vi "Maintain Loop Speed.vi"(7 "PID":T1={"proportional gain (Kc)"=10.0, "integral time (Ti, min)"=10.0, "derivative time (Td, min)"=0.0001}, 9 "setpoint (msec)":i32=25) -> (1 "Loop Time":dbl format="%0.2f")   [LabVIEW 2020]
uses:
  <vilib>/addons/control/pid/pid.llb/PID (DBL).vi
  <vilib>/ptbypt/NI_PtbyPt.lvlib
  <vilib>/addons/control/pid/NI_PID_pid.lvlib
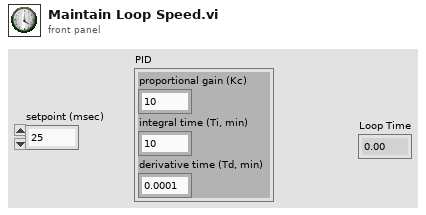
[diagram p1: front panel]
types:
  T1 = cluster{"proportional gain (Kc)":dbl, "integral time (Ti, min)":dbl, "derivative time (Td, min)":dbl}
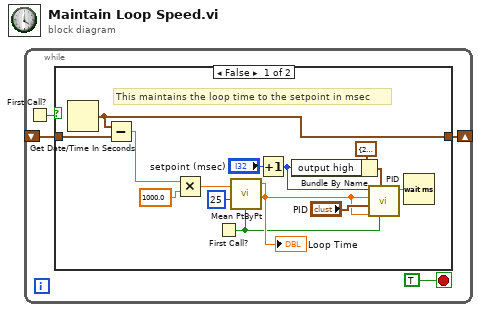
[diagram p0: block diagram]
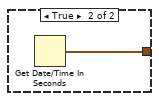
[diagram p2: hidden frame]
diagram:
  n1 = while {
    shift-right: [w2] -> _
    shift-left: _ -> [w3]
    stop <- TRUE stop-if-true
    n2 = First Call?() -> (First Call?: T/F=w1:bool)
    n3 = case shown="False" w1 {
      tunnel: w3 -> [w8 _]
      tunnel: [w7 w19] -> w2
      frame False {
        # "This maintains the loop time to the setpoint in msec"
        n4 = Get Date/Time In Seconds() -> (seconds since 1Jan1904=w7:timestamp)
        n5 = Subtract(x=w7, y=w8) -> (x-y=w6:dbl)
        n6 = Multiply(x=w6, y=1000.0) -> (x*y=w14:dbl)
        n7 = First Call?() -> (First Call?: T/F=w12:bool)
        n8 = call <vilib>:"Mean PtByPt.vi"("x"=w14, "sample length"=25, "initialize"=w12) -> ("mean"=w13:dbl)  [unwired: 1 in, 1 out]
        "Loop Time" <- w13
        n9 = Increment(x="setpoint (msec)") -> (x+1=w5:i32)
        n10 = Bundle By Name(cluster=cluster{"output high":dbl, "output low":dbl} {"output high"=25.0, "output low"=0.0} ("output range"), "output high"=w5) -> (w9:cluster{"output high":dbl, "output low":dbl})
        n11 = call-poly <vilib>:"PID.vi"("reinitialize? (F)"=w12, "output range"=w9, "dt (s)"=w13, "PID gains"="PID", "process variable"=w13, "setpoint"=w5) -> ("output"=w15:dbl)  [unwired: 4 in, 1 out]
        n12 = Wait (ms)(milliseconds to wait=w15) -> ()  [unwired: 1 out]
      }
      frame True {
        n13 = Get Date/Time In Seconds() -> (seconds since 1Jan1904=w19:timestamp)
      }
    }
  }
